vi "CLD 4 Event Structure Time Out Solution.vi"() -> ()   [LabVIEW 2009]
doc: "CLD-Übung 4\n\nDieses VI veranschaulicht die Verwendung des Timeout-Anschlusses der Ereignisstruktur."
panel:
  out "Zählwert":u32
  in  "Dekrementieren":bool
  out "Fehler (Ausgang)":T1
  in  "Fehler (Eingang)":T1
  out "Zeit ist verstrichen":bool
  in  "Inkrementieren":bool
  in  "VI anhalten":bool
  in  "Zielzeit (s)":dbl
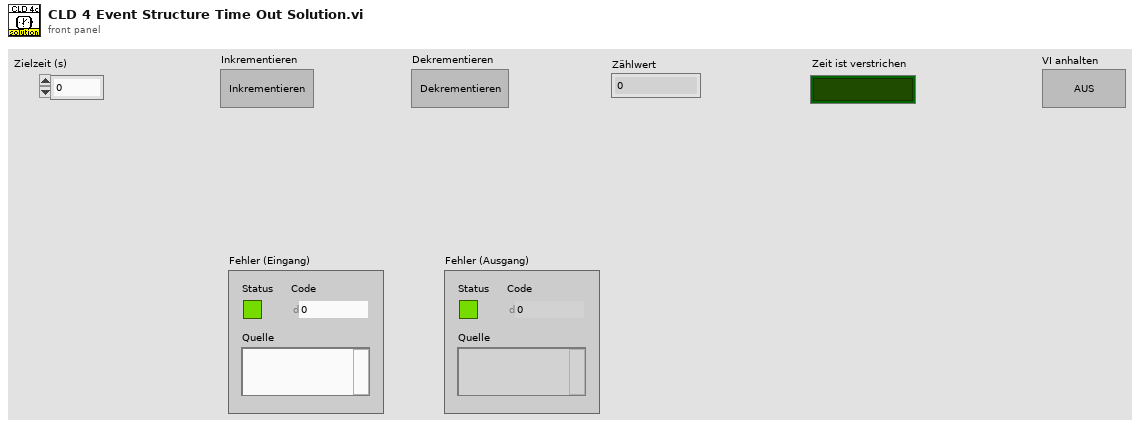
[diagram p1: front panel]
types:
  T1 = cluster{"Status":bool, "Code":i32, "Quelle":string}
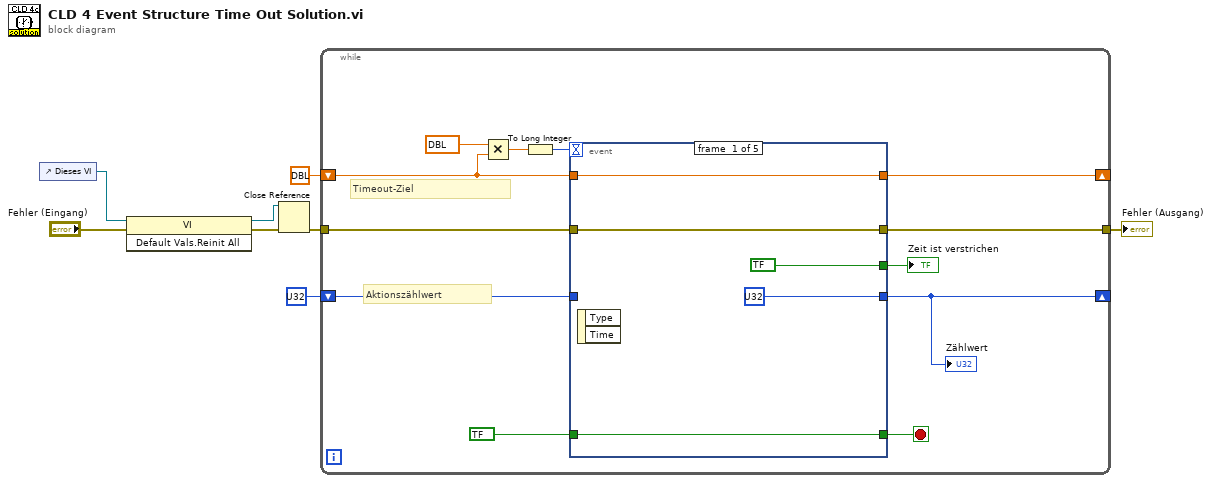
[diagram p0: block diagram]
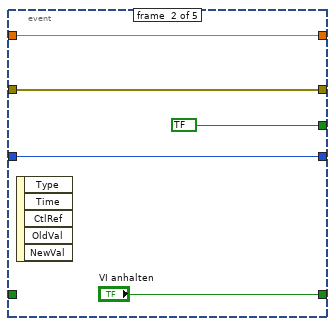
[diagram p2: hidden frame]
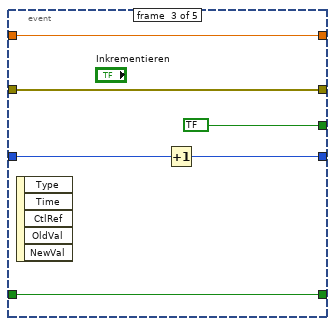
[diagram p3: hidden frame]
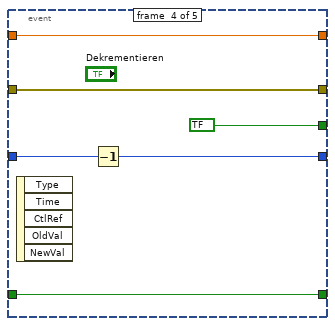
[diagram p4: hidden frame]
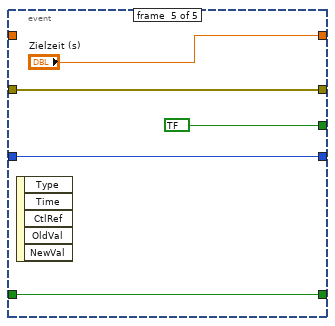
[diagram p5: hidden frame]
diagram:
  n1 = control-ref of="Dieses VI"() -> (w4:refnum<vi>)
  n2 = invoke class="VI" method="Default Vals.Reinit All"(reference=w4, error in="Fehler (Eingang)") -> (reference out=w2:refnum<vi>, error out=w5:errorcluster)  [unwired: 1 in, 1 out]
  n3 = Close Reference(reference=w2, error in (no error)=w5) -> (error out=w3:errorcluster)
  n4 = while {
    shift-right: [w15] -> _
    shift-left: u32 ? -> [w20]
    tunnel: w3 -> [w19]
    tunnel: [w18] -> w6
    shift-right: [w11] -> _
    shift-left: dbl ? ("Zielzeit (s)") -> [w10]
    stop <- w13 stop-if-true
    # "Aktionszählwert"
    # "Timeout-Ziel"
    n5 = Multiply(x=dbl ?, y=w10) -> (x*y=w14:dbl)
    n6 = To Long Integer(number=w14) -> (32bit integer=w9:i32)
    n7 = event shown="[4] \"Zielzeit (s)\": Value Change" {
      selector: _ -> [_ _ _ _ _]
      dyn-events: _ -> [_ _ _ _ _]
      timeout: w9 -> [_ _ _ _ _]
      tunnel: [u32 ? w26 w33 w40 w44] -> w15
      tunnel: w20 -> [_ w26 w34 w41 w44]
      tunnel: [bool ? bool ? bool ? bool ? bool ?] -> w16
      tunnel: w19 -> [w25 w30 w35 w42 w47]
      tunnel: [w25 w30 w35 w42 w47] -> w18
      tunnel: [w22 "VI anhalten" w32 w38 w46] -> w13
      tunnel: bool ? -> [w22 _ w32 w38 w46]
      tunnel: [w21 w28 w31 w37 "Zielzeit (s)"] -> w11
      tunnel: w10 -> [w21 w28 w31 w37 _]
      event #0 {
        n8 = event-data() -> ()  [unwired: 1 in, 2 out]
      }
      event #1 {
        n9 = event-data() -> ()  [unwired: 1 in, 5 out]
      }
      event #2 {
        n10 = event-data() -> ()  [unwired: 1 in, 5 out]
        n11 = Increment(x=w34) -> (x+1=w33:u32)
      }
      event #3 {
        n12 = event-data() -> ()  [unwired: 1 in, 5 out]
        n13 = Decrement(x=w41) -> (x-1=w40:u32)
      }
      event #4 {
        n14 = event-data() -> ()  [unwired: 1 in, 5 out]
      }
    }
    "Zeit ist verstrichen" <- w16
    "Zählwert" <- w15
  }
  "Fehler (Ausgang)" <- w6
